vi "serialito.vi"() -> ()   [LabVIEW 2018]
uses:
  <vilib>/Instr/_visa.llb/VISA Configure Serial Port (Instr).vi
panel:
  out "read buffer":string
  out "*(type *) &x":u16
  in  "stop":bool
  in  "baud rate (9600)":u32=9600
  in  "VISA resource name":refnum<visa-resource-name>
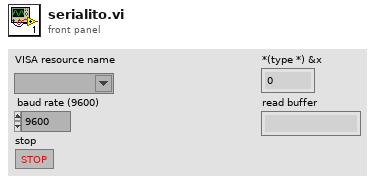
[diagram p1: front panel]
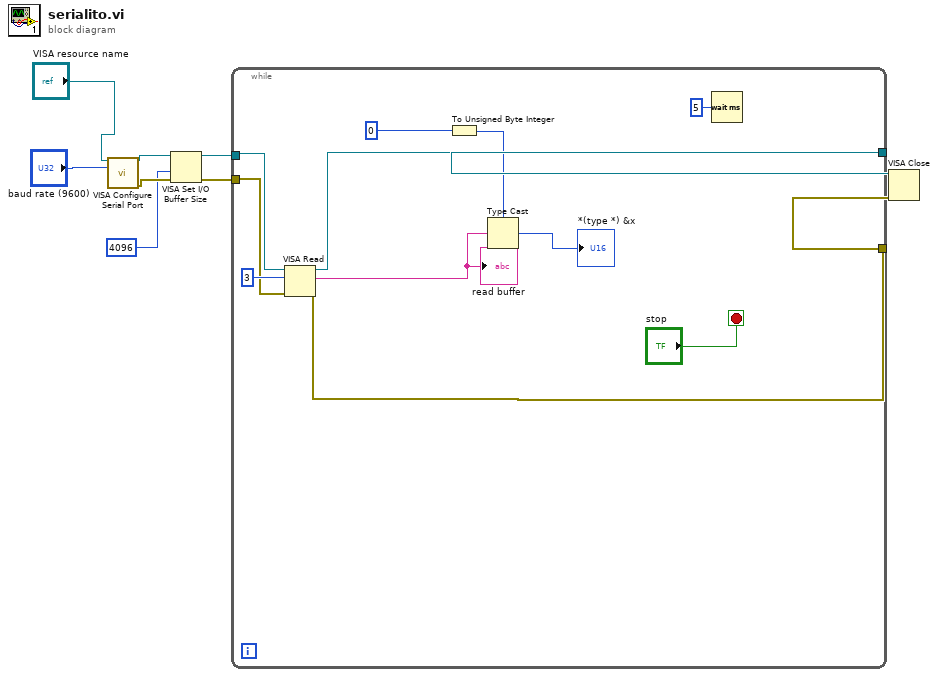
[diagram p0: block diagram]
diagram:
  n1 = call-poly "VISA Configure Serial Port"("VISA resource name"="VISA resource name", "baud rate (9600)"="baud rate (9600)") -> ("VISA resource name out"=w6:refnum<visa-resource-name>, "error out"=w4:errorcluster)  [unwired: 12 in]
  n2 = VISA Set I/O Buffer Size(VISA resource name=w6, size (4096)=u32 4096, error in (no error)=w4) -> (VISA resource name out=w5:refnum<visa-resource-name>, error out=w3:errorcluster)  [unwired: 1 in]
  n3 = while {
    tunnel: [w19] -> w8
    tunnel: w5 -> [w16]
    tunnel: w3 -> [w14]
    tunnel: [w13] -> w2
    stop <- "stop" stop-if-true
    n4 = VISA Read(VISA resource name=w16, byte count=u32 3, error in (no error)=w14) -> (VISA resource name out=w19:refnum<visa-resource-name>, read buffer=w10:string, error out=w13:errorcluster)  [unwired: 1 out]
    "read buffer" <- w10
    n5 = To Unsigned Byte Integer(number=u16 0) -> (unsigned 8bit integer=w12:u8)
    n6 = Type Cast(type=w12, x=w10) -> (*(type *) &x=→"*(type *) &x":u8)
    n7 = Wait (ms)(milliseconds to wait=u32 5) -> ()  [unwired: 1 out]
  }
  n8 = VISA Close(VISA resource name=w8, error in (no error)=w2) -> ()  [unwired: 1 out]
